vi "Get XY.vi"(8 "error in":errorcluster, 10 "Element Branch In":refnum<class "Tree.lvclass">, 11 "Element.lvclass In":refnum<class "Element.lvclass">) -> (0 "error out":errorcluster, 2 "Element Branch out":refnum<class "Tree.lvclass">, 3 "Element.lvclass Out":refnum<class "Element.lvclass">)   [LabVIEW 2019, in "ParseGDSII.lvclass"]
uses:
  ParseGDSII.lvclass
  Elements/Element.lvclass
  Tree/Tree.lvclass
  DataTypes/Base/GDSII.DataType.lvclass
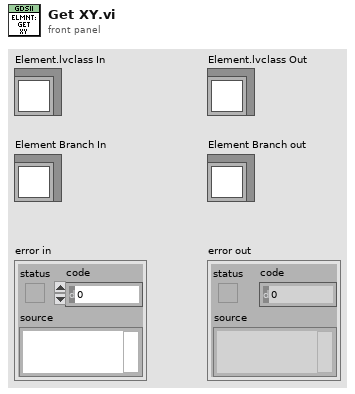
[diagram p1: front panel]
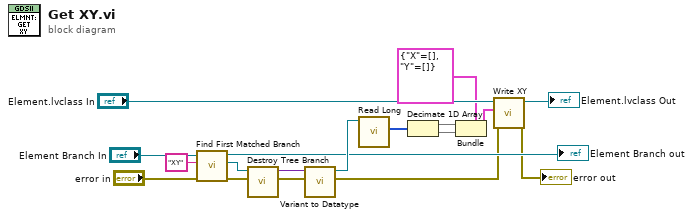
[diagram p0: block diagram]
diagram:
  n1 = call "Find First Matched Branch.vi"("error in"="error in", "Branch Name Exact"="XY", "Tree in"="Element Branch In") -> ("error out"=w10:errorcluster, "Matched Branch"=w17:refnum<class "Tree.lvclass">, "Tree out"=→"Element Branch out":refnum<class "Tree.lvclass">)  [unwired: 5 in, 1 out]
  n2 = call "Destroy Tree Branch.vi"("error in"=w10, "Tree in"=w17) -> ("error out"=w12:errorcluster, "Root"=w16:variant)  [unwired: 8 in]
  n3 = call "Variant to Datatype.vi"("error in"=w12, "Variant"=w16) -> ("error out"=w9:errorcluster, "DataType"=w15:refnum<class "GDSII.DataType.lvclass">)  [unwired: 8 in]
  n4 = call-dynamic "Read Long.vi"("GDSII.DataType in"=w15) -> ("Long"=w14:i32[])  [unwired: 9 in, 1 out]
  n5 = Decimate 1D Array(w14) -> (w2:i32[], w1:i32[])
  n6 = Bundle(cluster=cluster{"X":i32[], "Y":i32[]} {"X"=[], "Y"=[]} ("XY"), "X"=w2, "Y"=w1) -> (w11:cluster{"X":i32[], "Y":i32[]})
  n7 = call-dynamic "Write XY.vi"("error in (no error)"=w9, "XY"=w11, "Element in"="Element.lvclass In") -> ("error out"=→"error out":errorcluster, "Element out"=→"Element.lvclass Out":refnum<class "Element.lvclass">)  [unwired: 7 in]
